vi "JSON数据至数组转换.vi"(8 "error in (no error)":errorcluster caption="错误输入（无错误）", 11 "JSON数据":string) -> (0 "error out":errorcluster caption="错误输出", 2 "值":string[](array[string]), 3 "键":string[](array[string]))   [LabVIEW 2014]
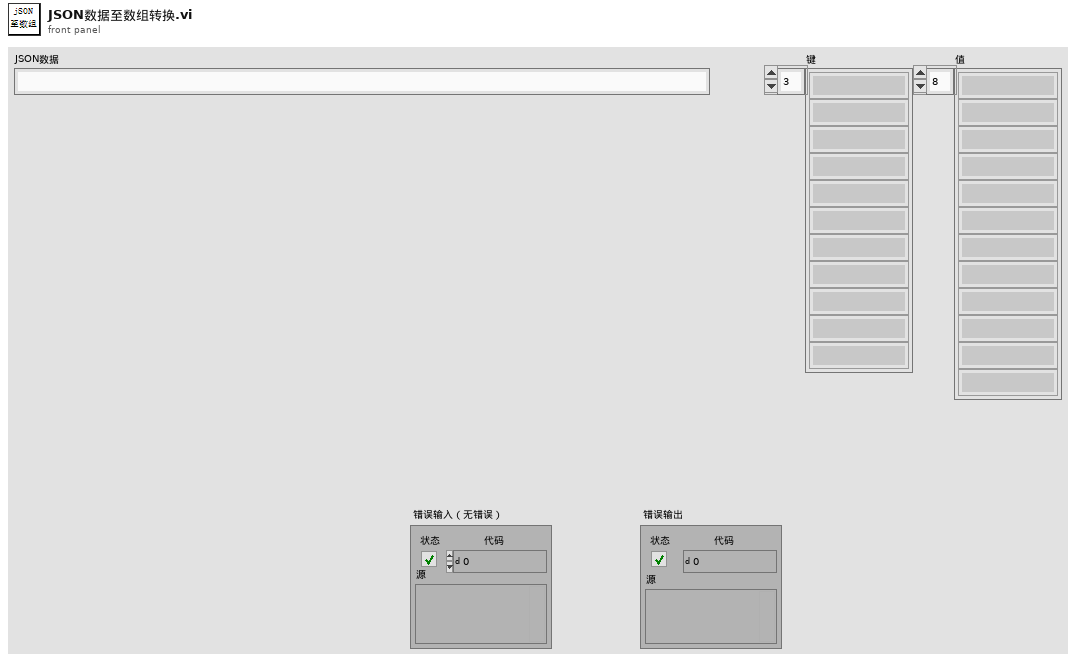
[diagram p1: front panel]
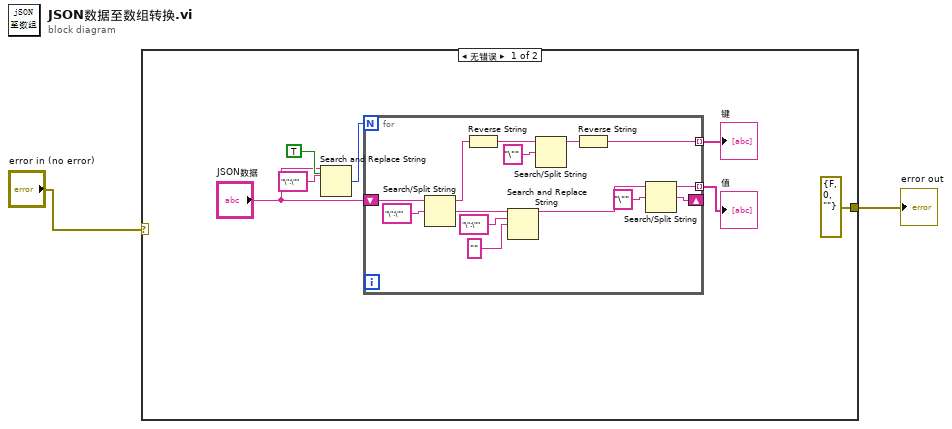
[diagram p0: block diagram]
diagram:
  n1 = case shown="无错误" "error in (no error)" {
    selector: "error in (no error)" -> [_ w24]
    tunnel: [errorcluster {"status"=FALSE, "code"=0, "source"=""} ("error IO") w24] -> w1
    frame No Error {
      n2 = Search and Replace String(replace all?=TRUE ("替换全部？(F)"), input string="JSON数据", search string="\":\"" ("搜索字符串")) -> (number of replacements=w6:i32)  [unwired: 5 in, 3 out]
      n3 = for {
        N: w6 -> [_]
        shift-right: [w12] -> _
        shift-left: "JSON数据" -> [w23]
        tunnel: [w11] -> w4 mode=indexing
        tunnel: [w10] -> w5 mode=indexing
        n4 = Search/Split String(string=w23, search string/char (-)="\":\"" ("搜索字符串")) -> (substring before match=w21:string, match + rest of string=w17:string)  [unwired: 1 in, 1 out]
        n5 = Reverse String(1:w21) -> (0:w20:string)
        n6 = Search and Replace String(input string=w17, search string="\":\"" ("搜索字符串"), replace string="" ("搜索字符串")) -> (result string=w15:string)  [unwired: 5 in, 3 out]
        n7 = Search/Split String(string=w20, search string/char (-)="\"" ("搜索字符串")) -> (substring before match=w19:string)  [unwired: 1 in, 2 out]
        n8 = Reverse String(1:w19) -> (0:w10:string)
        n9 = Search/Split String(string=w15, search string/char (-)="\"" ("搜索字符串")) -> (substring before match=w11:string, match + rest of string=w12:string)  [unwired: 1 in, 1 out]
      }
      "键" <- w5
      "值" <- w4
    }
    frame Error {
    }
  }
  "error out" <- w1
